vi "DriveModuleControl_TravTuneKa.vi"(8 "error in":errorcluster, 9 "Actual State":T1={"Speed"=0.0, "Angle"={"VALUE"=0.0, "COS"=1.0, "SIN"=0.0}} {"Angle"."SIN" format="%13.4f"; "Angle"."COS" format="%13.4f"; "Angle"."VALUE" format="%13.4f"}, 10 "Desired State":T1={"Speed"=0.0, "Angle"={"VALUE"=0.0, "COS"=1.0, "SIN"=0.0}} {"Angle"."SIN" format="%13.4f"; "Angle"."COS" format="%13.4f"; "Angle"."VALUE" format="%13.4f"}, 11 "ModualNamePrefix":i32) -> (0 "error out":errorcluster)   [LabVIEW 2023]
uses:
  <vilib>/Rock Robotics/WPI/ThirdParty/JAS_Junk/TrajLib/TypeDef/SWERVE_DRIVE_MODULE_STATE.ctl
  <vilib>/Rock Robotics/WPI/ThirdParty/JAS_Junk/TrajLib/TypeDef/ROTATION2D.ctl
  <vilib>/Rock Robotics/WPI/ThirdParty/JAS_Junk/TrajLib/Rotation2d_Minus.vi
  <vilib>/Rock Robotics/WPI/ThirdParty/JAS_Junk/TrajLib/Rotation2d_GetRadians.vi
  <vilib>/Rock Robotics/WPI/ThirdParty/JAS_Junk/TrajLib/SwerveModuleState_New.vi
  <vilib>/Rock Robotics/WPI/ThirdParty/JAS_Junk/TrajLib/Rotation2d_RotateBy.vi
  <vilib>/Rock Robotics/WPI/ThirdParty/JAS_Junk/TrajLib/Rotation2d_CreateAngle.vi
  <vilib>/Rock Robotics/WPI/ThirdParty/JAS_Junk/TrajLib/SimpleMotorFF_Calculate.vi
  <vilib>/Rock Robotics/WPI/ThirdParty/JAS_Junk/TrajLib/PIDController_AtSetpoint.vi
  <vilib>/Rock Robotics/WPI/ThirdParty/JAS_Junk/TrajLib/PIDController_SetPIDF.vi
  <vilib>/Rock Robotics/WPI/ThirdParty/JAS_Junk/TrajLib/PIDController_SetDerivativeFilter.vi
  <vilib>/Rock Robotics/WPI/ThirdParty/JAS_Junk/TrajLib/PIDController_SetIntegratorRange.vi
  <vilib>/Rock Robotics/WPI/ThirdParty/JAS_Junk/TrajLib/PIDController_SetTolerancePandV.vi
  <vilib>/Rock Robotics/WPI/ThirdParty/JAS_Junk/TrajLib/PIDController_DisableContinousInput.vi
  <vilib>/Rock Robotics/WPI/ThirdParty/JAS_Junk/TrajLib/PIDController_EnableContinousInput.vi
  <vilib>/Rock Robotics/WPI/ThirdParty/JAS_Junk/TrajLib/PIDController_Reset.vi
  <vilib>/Rock Robotics/WPI/ThirdParty/JAS_Junk/TrajLib/PIDController_New.vi
  <vilib>/Rock Robotics/WPI/ThirdParty/JAS_Junk/TrajLib/PIDController_SetOutputLimits.vi
  <vilib>/Rock Robotics/WPI/ThirdParty/JAS_Junk/TrajLib/Rotation2d_UnaryMinus.vi
  <vilib>/Rock Robotics/WPI/ThirdParty/JAS_Junk/TrajLib/Rotation2d_CreateXY.vi
  <vilib>/Rock Robotics/WPI/ThirdParty/JAS_Junk/TrajLib/PIDController_NewPeriod.vi
  <vilib>/Rock Robotics/WPI/ThirdParty/JAS_Junk/TrajLib/Util_CalcDist.vi
  <vilib>/Rock Robotics/SystemInterfaces/NetworkCommunication/NetComm_UsageReport_report.vi
  DriveGlobal.vi
  <vilib>/Rock Robotics/WPI/ThirdParty/JAS_Junk/TrajLib/Globals/Util_LibraryGlobals.vi
  <vilib>/Rock Robotics/WPI/ThirdParty/JAS_Junk/TrajLib/PIDController_AdvCalculate_FF_Sp_Pv.vi
  <vilib>/Rock Robotics/Network Tables/NT Write Number.vi
  <vilib>/Rock Robotics/Network Tables/NT Write Boolean.vi
  <vilib>/Rock Robotics/WPI/ThirdParty/JAS_Junk/TrajLib/Trajectory_Library.lvlib
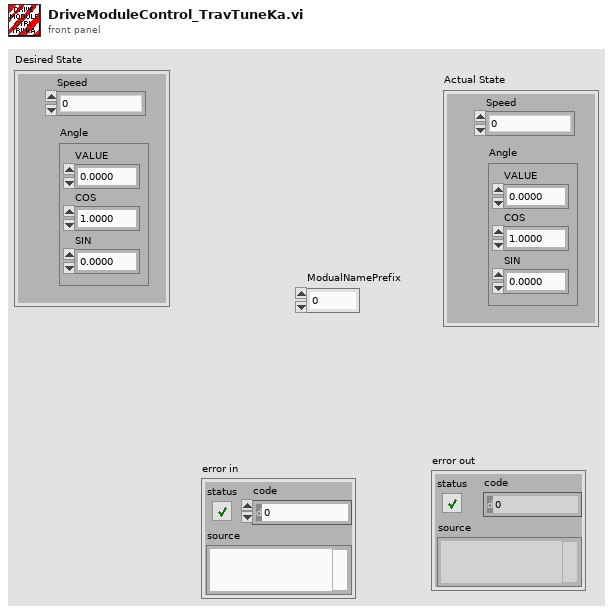
[diagram p1: front panel]
types:
  T1 = typedef "Trajectory_Library.lvlib/SWERVE_DRIVE_MODULE_STATE.ctl" = cluster{"Speed":dbl, "Angle":T2}
  T2 = typedef "Trajectory_Library.lvlib/ROTATION2D.ctl" = cluster{"VALUE":dbl, "COS":dbl, "SIN":dbl}
  T3 = typedef "WPI_MotorControlDeviceRef.ctl" = cluster{"DeviceStatus":errorcluster, "Type":T4, "PWM":cluster{"PWM Channel":T5, "DeadBand":T6}, "CAN":cluster{"Device Number":u8, "SetOutput VI Ref":variant, "GetOutput VI Ref":variant, "Enable VI Ref":variant, "Disable VI Ref":variant, "Data":variant}, "Invert":bool, "DIO PWM":cluster{"PWM \"Enable\" Channel":T5, "DIOChannel":T7, "PWM Rate":dbl}}
  T4 = typedef "WPI_MotorControlType.ctl" = enum16{"PWM", "CAN", "DIO PWM"}
  T5 = typedef "FPGA_DIOPWMChannel.ctl" = enum8{"PWM 0", "PWM 1", "PWM 2", "PWM 3", "PWM 4", "PWM 5", "PWM 6", "PWM 7", "PWM 8", "PWM 9", "PWM MXP 0", "PWM MXP 1", "PWM MXP 2", "PWM MXP 3", "PWM MXP 4", "PWM MXP 5", "PWM MXP 6", "PWM MXP 7", "PWM MXP 8", "PWM MXP 9", "Invalid"}
  T6 = typedef "WPI_PWMDeadband.ctl" = cluster{"Name":string, "maxPositivePwm":i32, "minPositivePwm":i32, "centerPwm":i32, "maxNegativePwm":i32, "minNegativePwm":i32, "angularRange":u16}
  T7 = typedef "FPGA_DIOChannel.ctl" = enum8{"DIO 0", "DIO 1", "DIO 2", "DIO 3", "DIO 4", "DIO 5", "DIO 6", "DIO 7", "DIO 8", "DIO 9", "DIO MXP 0", "DIO MXP 1", "DIO MXP 2", "DIO MXP 3", "DIO MXP 4", "DIO MXP 5", "DIO MXP 6", "DIO MXP 7", "DIO MXP 8", "DIO MXP 9", "DIO MXP 10", "DIO MXP 11", "DIO MXP 12", "DIO MXP 13", "DIO MXP 14", "DIO MXP 15", "SPI Port CS1", "SPI Port CS2", "SPI Port CS3", "SPI Port MISO", "SPI Port MOSI", "Invalid"}
  T8 = typedef "Trajectory_Library.lvlib/SIMPLE_MOTOR_FF.ctl" = cluster{"Ks":dbl, "Kv":dbl, "Ka":dbl, "KnInv":dbl}
  T9 = typedef "Trajectory_Library.lvlib/PID_ADV_LIMITS.ctl" = cluster{"MaxInput":dbl, "MinInput":dbl, "Continuous":bool, "MaxOutput":dbl, "MinOutput":dbl}
  T10 = typedef "Trajectory_Library.lvlib/PID_ADV_TUNING.ctl" = cluster{"Kf":dbl, "Kp":dbl, "Ki":dbl, "Kd":dbl, "MaximumIntegral":dbl, "MinimumIntegral":dbl, "Filter Derivative":bool}
  T11 = typedef "Trajectory_Library.lvlib/SIMPLE_MOTOR_FF_KA_TUNE_PARAMS.ctl" = cluster{"Max SP":dbl, "Min Eval SP":dbl, "Max Eval SP":dbl, "Ramp Rate":dbl}
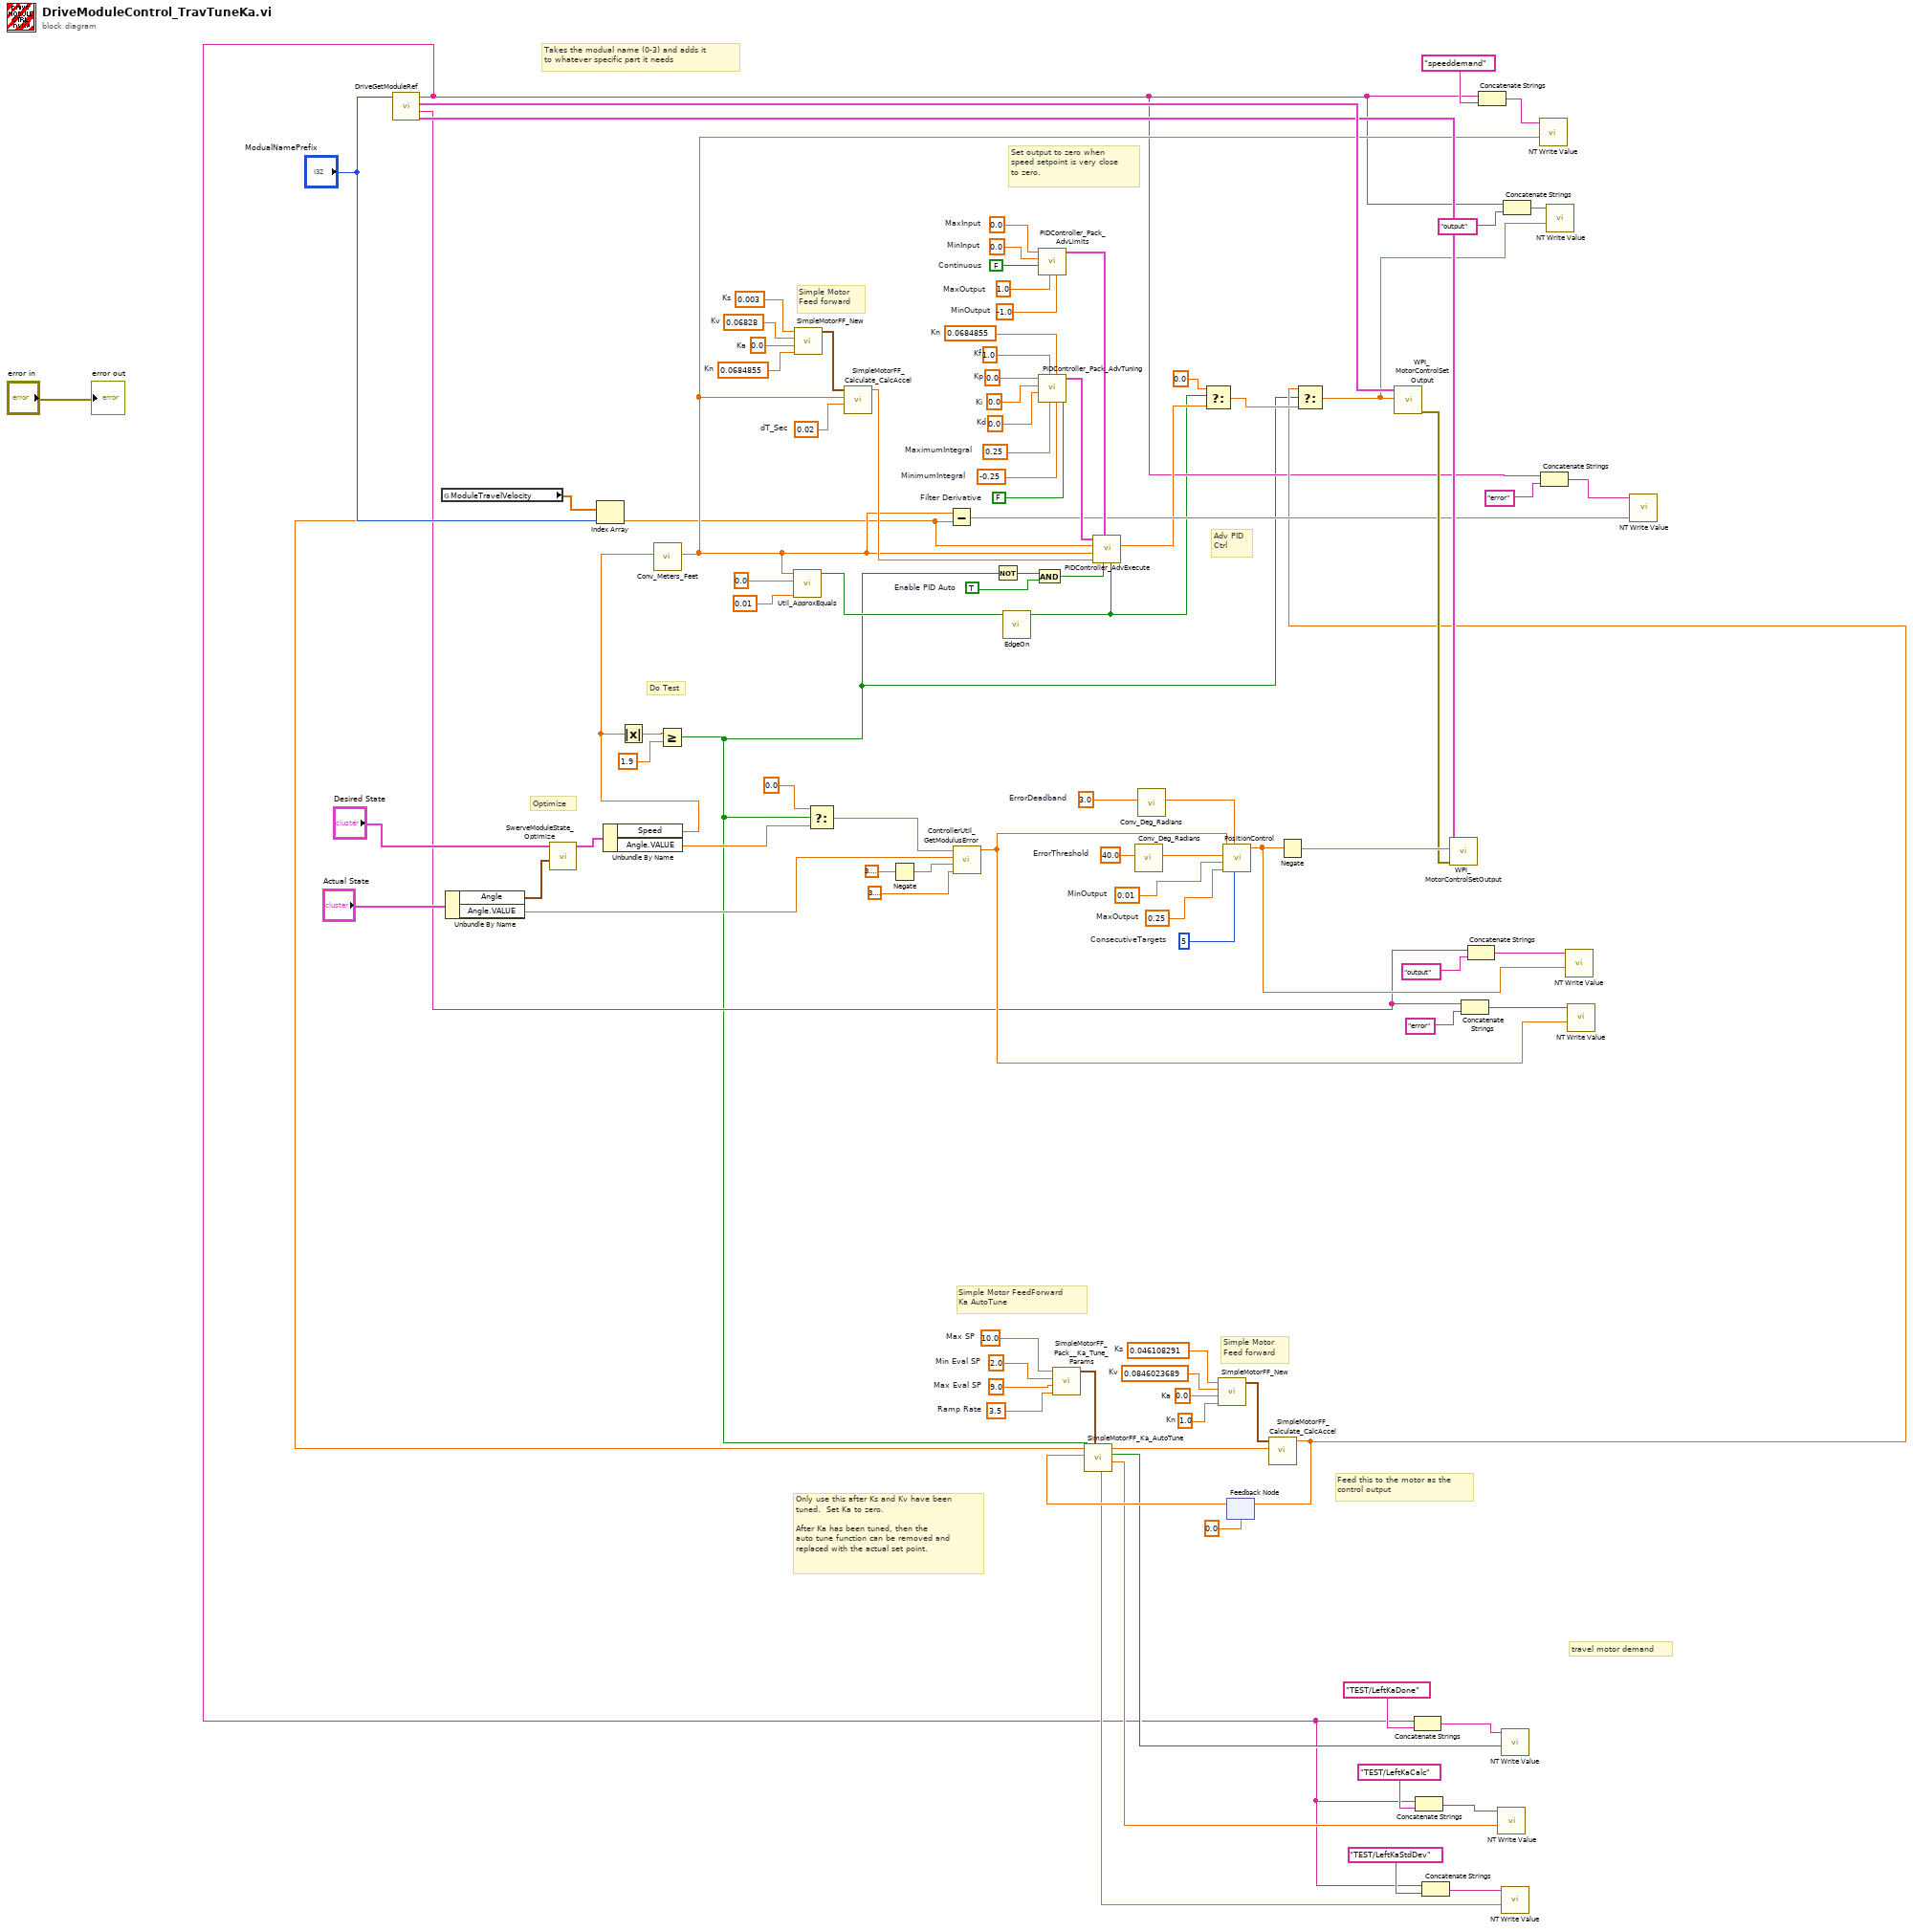
[diagram p0: block diagram]
diagram:
  w25 = 1.0  # Kn
  w23 = 0.046108291  # Ks
  w22 = 0.0846023689  # Kv
  w21 = 0.0  # Ka
  w20 = 10.0  # Max SP
  w19 = 2.0  # Min Eval SP
  w18 = 9.0  # Max Eval SP
  w17 = 3.5  # Ramp Rate
  w39 = TRUE  # Enable PID Auto
  w49 = 0.0684855  # Kn
  w66 = 0.0  # Kp
  w65 = 0.0  # Ki
  w64 = 0.0  # Kd
  w63 = 1.0  # Kf
  w62 = 0.25  # MaximumIntegral
  w61 = -0.25  # MinimumIntegral
  w60 = FALSE  # Filter Derivative
  w58 = 0.0  # MinInput
  w57 = FALSE  # Continuous
  w56 = 1.0  # MaxOutput
  w59 = -1.0  # MinOutput
  w55 = 0.0  # MaxInput
  w75 = 0.0684855  # Kn
  w74 = 0.02  # dT_Sec
  w72 = 0.003  # Ks
  w71 = 0.06828  # Kv
  w70 = 0.0  # Ka
  w85 = 5  # ConsecutiveTargets
  w82 = 0.25  # MaxOutput
  w86 = 0.01  # MinOutput
  w79 = 40.0  # ErrorThreshold
  w81 = 3.0  # ErrorDeadband
  # "Only use this after Ks and Kv have been\ntuned.  Set Ka to zero.\n\nAfter Ka has been tuned, then the \nauto tune function can be removed and\nreplaced with the actual set point."
  # "Feed this to the motor as the\ncontrol output"
  # "Simple Motor\nFeed forward"
  # "Simple Motor FeedForward\nKa AutoTune"
  # "travel motor demand"
  # "Do Test"
  # "Optimize"
  # "Set output to zero when\nspeed setpoint is very close\nto zero."
  # "Adv PID\nCtrl"
  # "Simple Motor\nFeed forward"
  # "Takes the modual name (0-3) and adds it \nto whatever specific part it needs"
  n1 = call "DriveGetModuleRef.vi"("ModualNamePrefix"="ModualNamePrefix") -> ("SpinMot"=w67:T3, "SpinStr"=w45:string, "TravMot"=w68:T3, "TravStr"=w4:string)  [unwired: 5 in, 2 out]
  n2 = global read "DriveGlobal.vi" "ModuleTravelVelocity"() -> (w51:dbl[])
  n3 = Unbundle By Name("Actual State") -> ("Angle"=w92:T2, "Angle.VALUE"=w89:dbl)
  n4 = call <vilib>:"SwerveModuleState_Optimize.vi"("CurrentAngle"=w92, "Desired State"="Desired State") -> ("out SWERVE_DRIVE_MODULE_STATE"=w90:T1)  [unwired: 9 in]
  n5 = Index Array(array=w51, index="ModualNamePrefix") -> (element=w12:dbl)
  n6 = Unbundle By Name(w90) -> ("Speed"=w36:dbl, "Angle.VALUE"=w33:dbl)
  n7 = Absolute Value(x=w36) -> (abs(x)=w35:dbl)
  n8 = call <vilib>:"Conv_Meters_Feet.vi"("Meters"=w36) -> ("Feet"=w42:dbl)  [unwired: 10 in]
  n9 = Greater Or Equal?(x=w35, y=1.9) -> (x >= y?=w1:bool)
  n10 = call <vilib>:"Util_ApproxEquals.vi"("Tolerance"=0.01, "Value 2"=0.0, "Value 1"=w42) -> ("ApproxEquals"=w3:bool)  [unwired: 8 in]
  n11 = call <vilib>:"SimpleMotorFF_New.vi"("Kn"=w75, "Ka"=w70, "Kv"=w71, "Ks"=w72) -> ("SIMPLE_MOTOR_FF"=w73:T8)  [unwired: 7 in]
  n12 = Select(t=0.0, s=w1, f=w33) -> (s? t:f=w29:dbl)
  n13 = call <vilib>:"SimpleMotorFF_Calculate_CalcAccel.vi"("dT_Sec"=w74, "VelSp"=w42, "SIMPLE_MOTOR_FF"=w73) -> ("FeedForward"=w52:dbl)  [unwired: 8 in]
  n14 = Negate(x=3.141592653589793) -> (-x=w91:dbl)
  n15 = Subtract(x=w42, y=w12) -> (x-y=w46:dbl)
  n16 = call <vilib>:"ControllerUtil_GetModulusError.vi"("Maximum_Input"=3.141592653589793, "Minimum_Input"=w91, "Measurerment(PV)"=w89, "Reference(SP)"=w29) -> ("Error"=w83:dbl)  [unwired: 7 in]
  n17 = Not(x=w1) -> (.not. x?=w40:bool)
  n18 = call "EdgeOn.vi"("Current State"=w3) -> ("Edge On Found"=w2:bool)  [unwired: 10 in]
  n19 = And(x=w40, y=w39) -> (x .and. y?=w41:bool)
  n20 = call <vilib>:"PIDController_Pack_AdvLimits.vi"("MinOutput"=w59, "MaxOutput"=w56, "Continuous"=w57, "MinInput"=w58, "MaxInput"=w55) -> ("Adv PID Limits"=w53:T9)  [unwired: 6 in]
  n21 = call <vilib>:"PIDController_Pack_AdvTuning.vi"("Filter Derivative"=w60, "MinimumIntegral"=w61, "Kn"=w49, "MaximumIntegral"=w62, "Kf"=w63, "Kd"=w64, "Ki"=w65, "Kp"=w66) -> ("Adv PID Tuning"=w54:T10)  [unwired: 3 in]
  n22 = call <vilib>:"SimpleMotorFF_Pack__Ka_Tune_Params.vi"("Ramp Rate"=w17, "Max Eval SP"=w18, "Min Eval SP"=w19, "Max SP"=w20) -> ("Packed Params"=w16:T11)  [unwired: 7 in]
  n23 = call <vilib>:"PIDController_AdvExecute.vi"("Reset"=w2, "Auto"=w41, "Adv PID Limits"=w53, "FF-FeedForward"=w52, "SP-SetPoint"=w42, "PV-Measurement"=w12, "Adv PID Tuning"=w54) -> ("CO-ControlOutput"=w38:dbl)  [unwired: 2 in, 2 out]
  n24 = call <vilib>:"Conv_Deg_Radians.vi"("Degress"=w79) -> ("Radians"=w78:dbl)  [unwired: 10 in]
  n25 = call <vilib>:"Conv_Deg_Radians.vi"("Degress"=w81) -> ("Radians"=w80:dbl)  [unwired: 10 in]
  n26 = Select(t=0.0, s=w2, f=w38) -> (s? t:f=w30:dbl)
  n27 = call <vilib>:"SimpleMotorFF_New.vi"("Kn"=w25, "Ka"=w21, "Kv"=w22, "Ks"=w23) -> ("SIMPLE_MOTOR_FF"=w24:T8)  [unwired: 7 in]
  n28 = call "PositionControl.vi"("ConsecutiveTargets"=w85, "ErrorDeadband"=w80, "MaxOutput"=w82, "MinOutput"=w86, "ErrorThreshold"=w78, "Error"=w83) -> ("OutputValue"=w77:dbl)  [unwired: 3 in, 2 out]
  n29 = feedback #1(0.0 ("FeedForward")) -> (w27:dbl)
  n30 = call <vilib>:"SimpleMotorFF_Ka_AutoTune.vi"("SimpleMotorFeedforward_KaTune_Pack"=w16, "Run Test"=w1, "CO Control Output"=w27, "PV ProcessVariable"=w12) -> ("Ka Calc"=w14:dbl, "Test Complete"=w15:bool, "SP Setpoint"=w26:dbl, "Ka StdDev"=w13:dbl)  [unwired: 1 in, 3 out]
  n31 = call <vilib>:"SimpleMotorFF_Calculate_CalcAccel.vi"("VelSp"=w26, "SIMPLE_MOTOR_FF"=w24) -> ("FeedForward"=w11:dbl)  [unwired: 9 in]
  n32 = feedback-in #1(w11) -> ()
  n33 = Negate(x=w77) -> (-x=w76:dbl)
  n34 = Select(t=w11, s=w1, f=w30) -> (s? t:f=w31:dbl)
  n35 = call <vilib>:"WPI_MotorControlSetOutput.vi"("Output"=w31, "MotorControlDevRef"=w68) -> ("error out"=w69:errorcluster)  [unwired: 7 in, 2 out]
  n36 = Concatenate Strings(w4, "TEST/LeftKaDone" ("name")) -> (w7:string)
  n37 = Concatenate Strings(w4, "TEST/LeftKaCalc" ("name")) -> (w6:string)
  n38 = Concatenate Strings(w4, "TEST/LeftKaStdDev" ("name")) -> (w5:string)
  n39 = call <vilib>:"WPI_MotorControlSetOutput.vi"("error in (no error)"=w69, "Output"=w76, "MotorControlDevRef"=w67) -> ()  [unwired: 6 in, 3 out]
  n40 = Concatenate Strings(w45, "error" ("refnum name")) -> (w96:string)
  n41 = Concatenate Strings(w45, "output" ("refnum name")) -> (w84:string)
  n42 = Concatenate Strings(w4, "speeddemand" ("refnum name")) -> (w100:string)
  n43 = call-poly <vilib>:"NT Write Value.vi"("value"=w14, "name"=w6) -> ()  [unwired: 9 in, 1 out]
  n44 = call-poly <vilib>:"NT Write Value.vi"("value"=w15, "name"=w7) -> ()  [unwired: 9 in, 1 out]
  n45 = call-poly <vilib>:"NT Write Value.vi"("value"=w13, "name"=w5) -> ()  [unwired: 9 in, 1 out]
  n46 = Concatenate Strings(w4, "output" ("refnum name")) -> (w98:string)
  n47 = call-poly <vilib>:"NT Write Value.vi"("value"=w42, "name"=w100) -> ()  [unwired: 9 in, 1 out]
  n48 = Concatenate Strings(w4, "error" ("refnum name")) -> (w47:string)
  n49 = call-poly <vilib>:"NT Write Value.vi"("value"=w31, "name"=w98) -> ()  [unwired: 9 in, 1 out]
  n50 = call-poly <vilib>:"NT Write Value.vi"("value"=w77, "name"=w84) -> ()  [unwired: 9 in, 1 out]
  n51 = call-poly <vilib>:"NT Write Value.vi"("value"=w83, "name"=w96) -> ()  [unwired: 9 in, 1 out]
  n52 = call-poly <vilib>:"NT Write Value.vi"("value"=w46, "name"=w47) -> ()  [unwired: 9 in, 1 out]
  "error out" <- "error in"
